vi "Write IL Action Override.vi"(10 "IL Action Override":refnum<class "IL Action.lvclass">[](array[class]), 11 "Interlock Chain in":refnum<class "Interlock Chain.lvclass">) -> (3 "Interlock Chain out":refnum<class "Interlock Chain.lvclass">)   [LabVIEW 2015, in "Interlocks.lvlib" / "Interlock Chain.lvclass"]
uses:
  Interlock Chain.lvclass
  IL Action/IL Action.lvclass
  Interlock Chain.lvclass/Interlock Chain.ctl
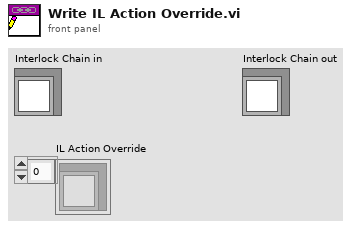
[diagram p1: front panel]
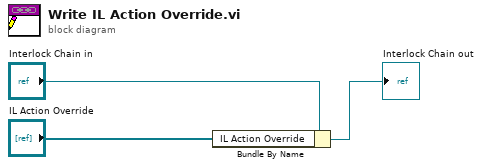
[diagram p0: block diagram]
diagram:
  n1 = Bundle By Name(cluster="Interlock Chain in", "IL Action Override"="IL Action Override") -> (→"Interlock Chain out":refnum<class "Interlock Chain.lvclass">)
